vi "DrawBuoy.vi"(2 "Array":dbl[][](array[numeric]), 3 "2D Picture":picture) -> (0 "new picture":picture)   [LabVIEW 2012]
doc: "Draws a magenta circle at the curretn (x,y) coordinates of the Robot in the current mission definition file.\nInputs:\nPicture to draw on\nCluster X\n y coordinates of robot\nOutput:\nmodified picture"
panel:
  # "Draws a circle at the current x,y coordinates of the robot"
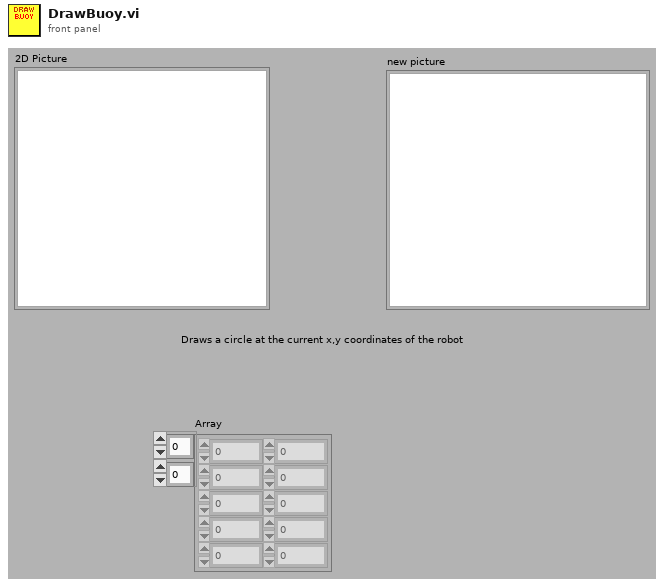
[diagram p1: front panel]
types:
  T1 = cluster{"Width":u16, "Style":enum32{"Solid", "Dash", "Dot", "DashDot", "DashDotDot"}}
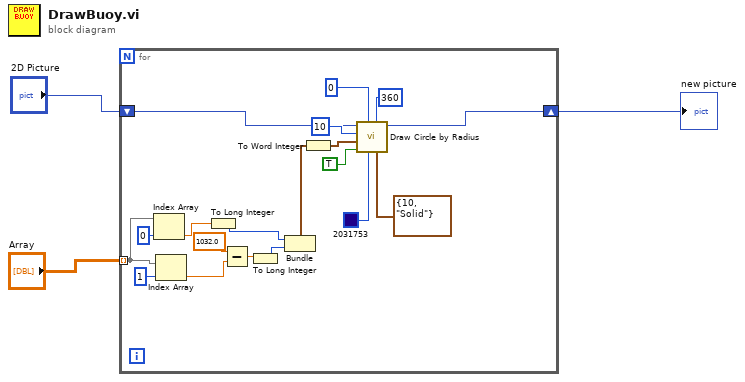
[diagram p0: block diagram]
diagram:
  n1 = for {
    shift-right: [w9] -> w2
    shift-left: "2D Picture" -> [w16]
    tunnel: "Array" -> [w6] mode=indexing
    n2 = Index Array(array=w6, index=0) -> (element=w4:dbl)
    n3 = Index Array(array=w6, index=1) -> (element=w5:dbl)
    n4 = To Long Integer(number=w4) -> (32bit integer=w13:i32)
    n5 = Subtract(x=1032.0, y=w5) -> (x-y=w12:dbl)
    n6 = To Long Integer(number=w12) -> (32bit integer=w11:i32)
    n7 = Bundle(w13, w11) -> (w10:cluster{i32, i32})  [unwired: 1 in]
    n8 = To Word Integer(number=w10) -> (16bit integer=w22:cluster{i16, i16})
    n9 = call <vilib>:"Draw Circle by Radius.vi"("pen"=T1 {"Width"=10, "Style"=enum."Solid"}, "arc size(360)"=i16 360, "color(black)"=u32 2031753, "start angle(0)"=i16 0, "fill?(F)"=TRUE, "pixel center"=w22, "radius"=i16 10, "picture"=w16) -> ("new picture"=w9:picture)  [unwired: 3 in]
  }
  "new picture" <- w2
